vi "LVClass_HasoSlopes NewFromXMLStringFormat.vi"(0 "HasoSlopes in":refnum<class "HasoSlopes.lvclass">, 5 "XML txt format":string="HAS xml txt format", 11 "error in (no error)":errorcluster) -> (4 "HasoSlopes out":refnum<class "HasoSlopes.lvclass">, 15 "error out":errorcluster)   [LabVIEW 2020, in "HasoSlopes.lvclass"]
doc: "int32_t ImOp_new_HasoSlopes_From_HAS_file(CStr message, int32_t *objet, const CStr chemin_config);"
uses:
  HasoSlopes.lvclass
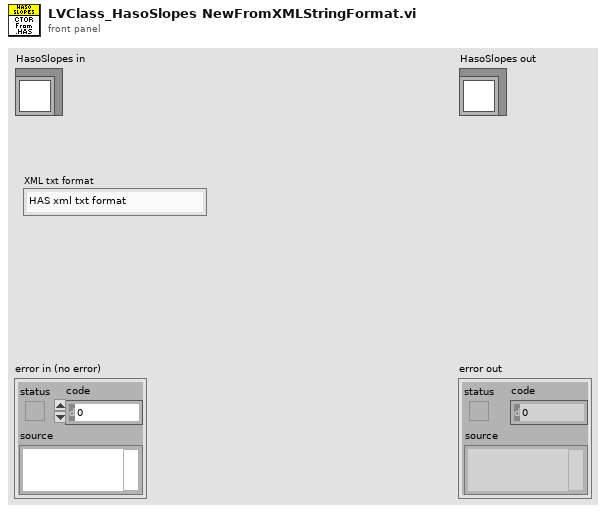
[diagram p1: front panel]
types:
  T1 = cluster{"second":i32, "minute":i32, "hour":i32, "day of month":i32, "month":i32, "year":i32, "day of week":i32, "day of year":i32, "is DST":i32}
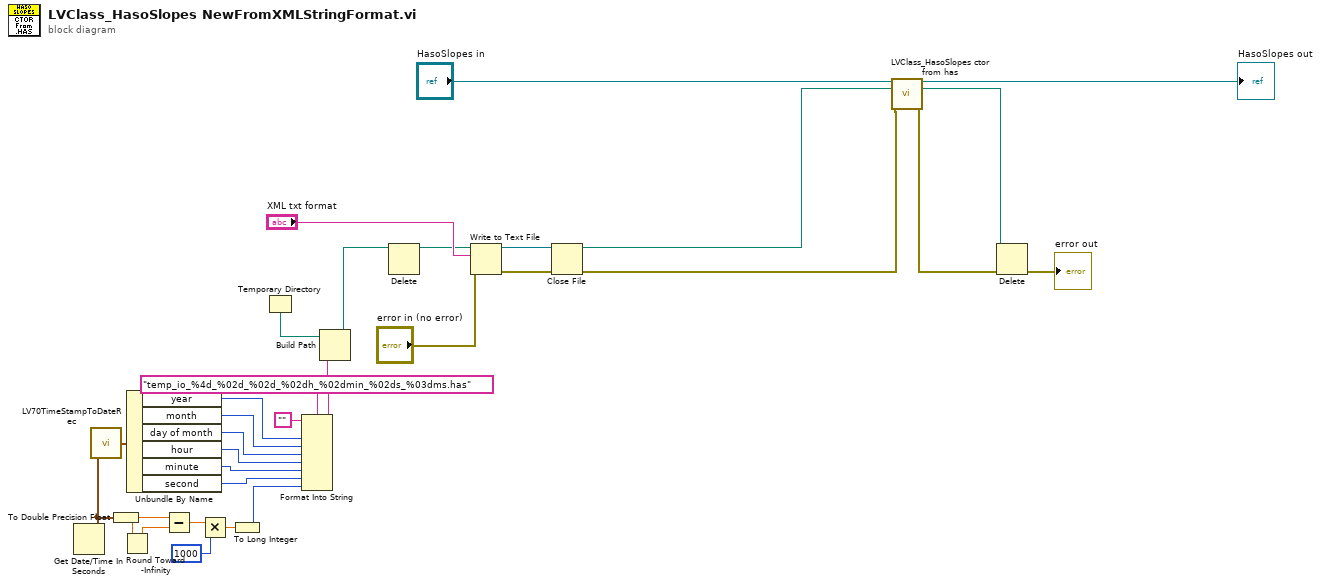
[diagram p0: block diagram]
diagram:
  n1 = Get Date/Time In Seconds() -> (seconds since 1Jan1904=w28:timestamp)
  n2 = call "LV70TimeStampToDateRec.vi"("time stamp"=w28) -> ("date time rec"=w29:T1)
  n3 = To Double Precision Float(number=w28) -> (double precision float=w27:dbl)
  n4 = Round Toward -Infinity(1:w27) -> (0:w26:dbl)
  n5 = Unbundle By Name(w29) -> ("year"=w19:i32, "month"=w20:i32, "day of month"=w18:i32, "hour"=w17:i32, "minute"=w16:i32, "second"=w15:i32)
  n6 = Subtract(x=w27, y=w26) -> (x-y=w25:dbl)
  n7 = Multiply(x=w25, y=1000) -> (x*y=w23:dbl)
  n8 = To Long Integer(number=w23) -> (32bit integer=w14:i32)
  n9 = Temporary Directory() -> (w30:path)
  n10 = Format Into String(format string="temp_io_%4d_%02d_%02d_%02dh_%02dmin_%02ds_%03dms.has", initial string="", w19, w20, w18, w17, w16, w15, w14) -> (resulting string=w13:string)  [unwired: 1 in, 1 out]
  n11 = Build Path(base path=w30, name or relative path=w13) -> (appended path=w12:path)
  n12 = Delete(path (use dialog)=w12) -> (deleted path=w5:path)  [unwired: 4 in, 2 out]
  n13 = Write to Text File(file (use dialog)=w5, text="XML txt format", error in="error in (no error)") -> (refnum out=w7:refnum<file>, error out=w6:errorcluster)  [unwired: 1 in, 1 out]
  n14 = Close File(refnum=w7, error in=w6) -> (path=w1:path, error out=w4:errorcluster)
  n15 = call "LVClass_HasoSlopes ctor from has.vi"("HasoSlopes (const)"="HasoSlopes in", ".has path"=w1, "error in (no error)"=w4) -> ("HasoSlopes (new)"=→"HasoSlopes out":refnum<class "HasoSlopes.lvclass">, "error out"=w3:errorcluster)  [unwired: 11 in]
  n16 = Delete(path (use dialog)=w1, error in=w3) -> (error out=→"error out":errorcluster)  [unwired: 3 in, 2 out]
